vi "ConfigEnbRead.vi"(2 "Read voltage? (n)":bool, 4 "Enable Output (T: Enable)":bool=TRUE, 5 "Config Voltage? (y)":bool=TRUE, 6 "Config Curr Limit? (n)":bool, 7 "Reset when done? (n)":bool, 8 "error in (no error)":errorcluster, 9 "Current Limit (amps)":dbl format="%.2f", 10 "Voltage (vdc)":dbl format="%.2f", 11 "VISA resource name":refnum<visa-resource-name>="Keith2200") -> (0 "error out":errorcluster, 1 "Voltage":string, 3 "VISA resource name out":refnum<visa-resource-name>)   [LabVIEW 2013]
uses:
  Keithley 2200 Series.lvlib
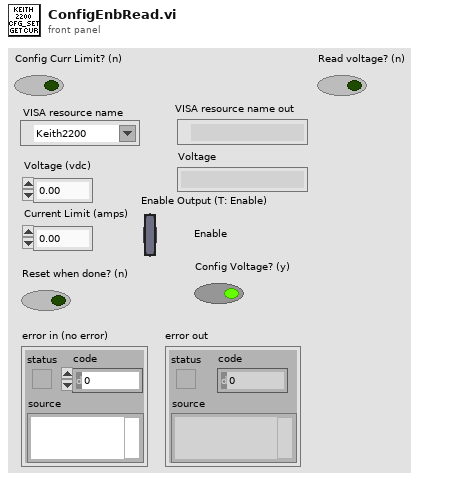
[diagram p1: front panel]
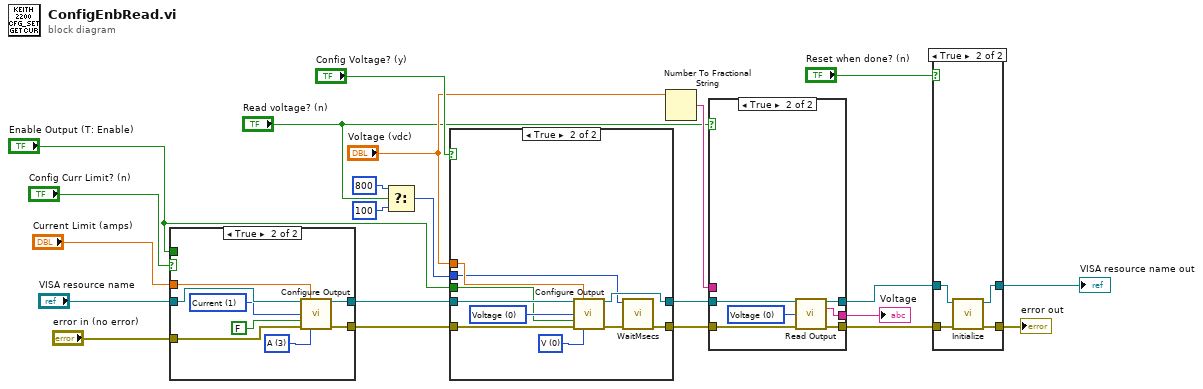
[diagram p0: block diagram]
diagram:
  n1 = case shown="True" "Config Curr Limit? (n)" {
    tunnel: "error in (no error)" -> [w24 w32]
    tunnel: "VISA resource name" -> [w23 w31]
    tunnel: [w24 w27] -> w12
    tunnel: [w23 w26] -> w11
    tunnel: "Current Limit (amps)" -> [_ w28]
    tunnel: "Enable Output (T: Enable)" -> [_ _]
    frame False {
    }
    frame True {
      w29 = u16 3 items=["V", "mV", "kV", "A", "mA"] ("Unit(V)")
      w30 = u16 1 items=["Voltage", "Current"] ("Function(0:Voltage)")
      n2 = call "Configure Output.vi"("VISA resource name"=w31, "Manual Range(0.00)"=w28, "Function(0:Voltage)"=w30, "Enable Output (T: Enable)"=FALSE, "error in (no error)"=w32, "Unit(V)"=w29) -> ("VISA resource name out"=w26:refnum<visa-resource-name>, "error out"=w27:errorcluster)  [unwired: 8 in]
    }
  }
  n3 = Select(t=u32 800 ("Wait Msecs"), s="Read voltage? (n)", f=u32 100 ("Wait Msecs")) -> (s? t:f=w1:u32)
  n4 = case shown="True" "Config Voltage? (y)" {
    tunnel: w12 -> [w34 w38]
    tunnel: w11 -> [w33 w37]
    tunnel: [w34 w42] -> w10
    tunnel: [w33 w41] -> w9
    tunnel: "Voltage (vdc)" -> [_ w39]
    tunnel: "Enable Output (T: Enable)" -> [_ w36]
    tunnel: w1 -> [_ w35]
    frame False {
    }
    frame True {
      w40 = u16 0 items=["Voltage", "Current"] ("Function(0:Voltage)")
      w43 = u16 0 items=["V", "mV", "kV", "A", "mA"] ("Unit(V)")
      n5 = call "Configure Output.vi"("VISA resource name"=w37, "Manual Range(0.00)"=w39, "Function(0:Voltage)"=w40, "Enable Output (T: Enable)"=w36, "error in (no error)"=w38, "Unit(V)"=w43) -> ("VISA resource name out"=w41:refnum<visa-resource-name>, "error out"=w44:errorcluster)  [unwired: 8 in]
      n6 = call "WaitMsecs.vi"("error in (no error)"=w44, "Wait Msecs"=w35) -> ("error out"=w42:errorcluster)  [unwired: 9 in]
    }
  }
  n7 = Number To Fractional String(number="Voltage (vdc)") -> (F-format string=w5:string)  [unwired: 3 in]
  n8 = case shown="True" "Read voltage? (n)" {
    tunnel: [w45 w52] -> w16
    tunnel: [w47 w51] -> w15
    tunnel: [w46 w50] -> w14
    tunnel: w10 -> [w47 w49]
    tunnel: w9 -> [w46 w48]
    tunnel: w5 -> [w45 _]
    frame False {
    }
    frame True {
      w53 = u16 0 items=["Voltage", "Current", "Power"] ("Measurement Function (0:Voltage)")
      n9 = call "Read Output.vi"("VISA resource name"=w48, "Measurement Function (0:Voltage)"=w53, "error in (no error)"=w49) -> ("VISA resource name out"=w50:refnum<visa-resource-name>, "Measurement"=w52:string, "error out"=w51:errorcluster)  [unwired: 10 in]
    }
  }
  "Voltage" <- w16
  n10 = case shown="True" "Reset when done? (n)" {
    tunnel: w15 -> [w55 w59]
    tunnel: w14 -> [w54 w58]
    tunnel: [w55 w57] -> w20
    tunnel: [w54 w56] -> w19
    frame False {
    }
    frame True {
      n11 = call "Initialize.vi"("error in (no error)"=w59, "VISA resource name"=w58) -> ("error out"=w57:errorcluster, "VISA resource name out"=w56:refnum<visa-resource-name>)  [unwired: 8 in]
    }
  }
  "VISA resource name out" <- w19
  "error out" <- w20
